vi "Test My Cloneable Module API.vi"() -> ()   [LabVIEW 2020]
doc: "My Module API Tester.\n_____\nBased on Delacor QMH Project Template 5.0.0.82."
uses:
  My Cloneable Module.lvlib
panel:
  in  "wait for reply":bool=TRUE
  in  "Run as Singleton?":bool
  in  "Show Block Diagram":bool
  in  "Refresh Modules":bool
  in  "X":dbl=1.0
  out "Reply Payload":dbl
  out "Active Modules":string[](array[string])
  in  "Stop Module":bool
  in  "Select Module":i32(ring)=-1 caption="Select Module\nTo send Request to" items=["All"=-1]
  in  "Run New Module":bool
  out "Do Something Count":i32
  in  "Test Do Something Else and Wait for Reply":bool
  in  "Hide Module Panel":bool
  in  "Show Module Panel":bool
  in  "Test Do Something Else":bool
  in  "Test Do Something":bool
  out "Status":string
  # "This VI tests the API for the Module."
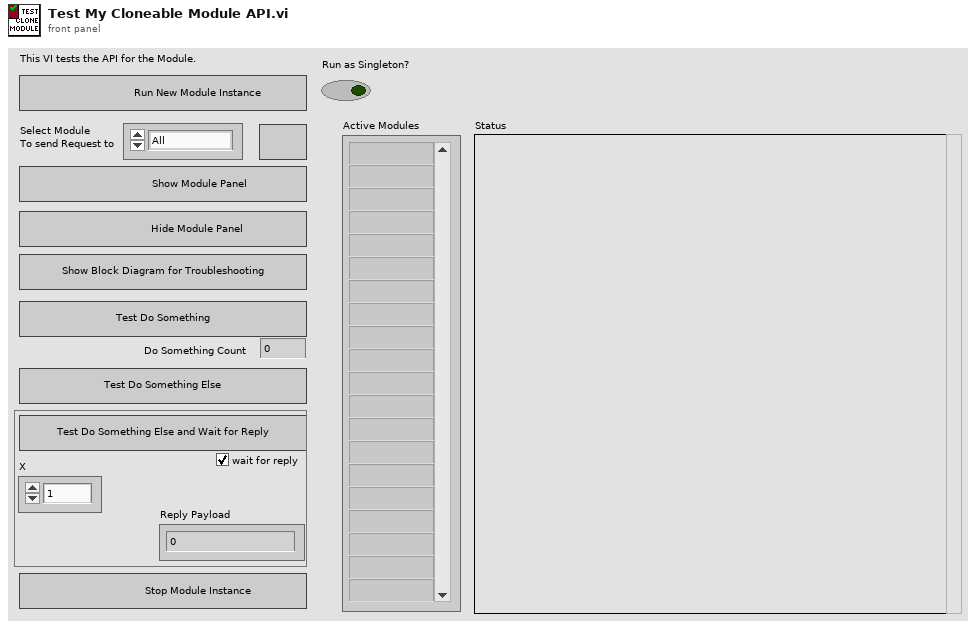
[diagram p1: front panel]
types:
  T1 = typedef "My Cloneable Module.lvlib/Broadcast Events--cluster.ctl" = cluster{"Module Did Init":refnum<user-event>, "Status Updated":refnum<user-event>, "Error Reported":refnum<user-event>, "Did Something":refnum<user-event>, "Module Did Stop":refnum<user-event>, "Update Module Execution Status":refnum<user-event>}
  T2 = typedef "My Cloneable Module.lvlib/Do Something Else and Wait (Reply Payload)--cluster.ctl" = cluster{"Value":dbl, "error":errorcluster}
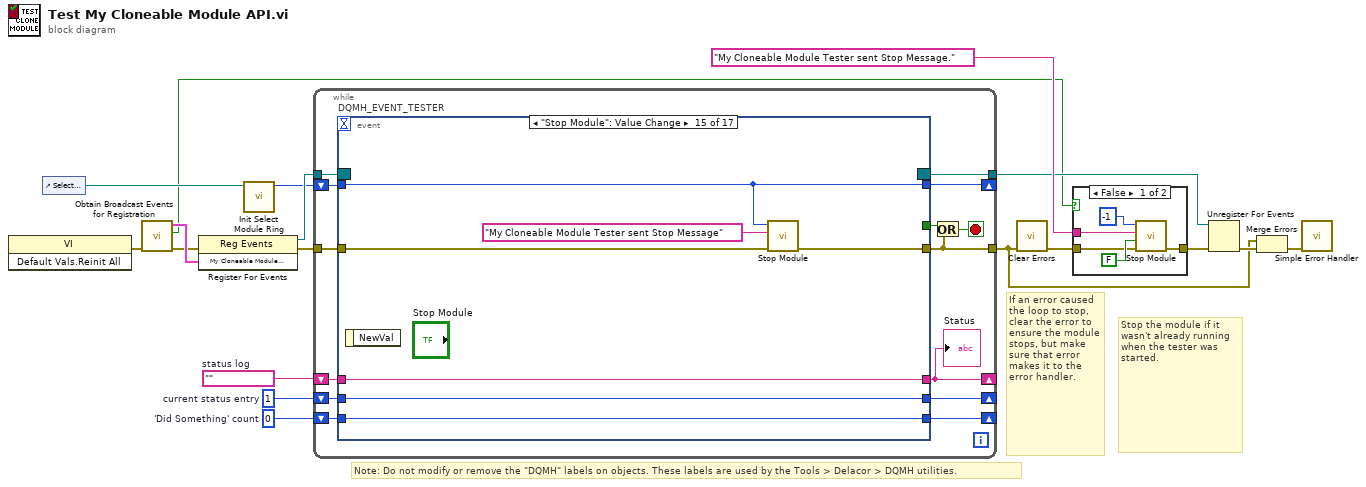
[diagram p0: block diagram]
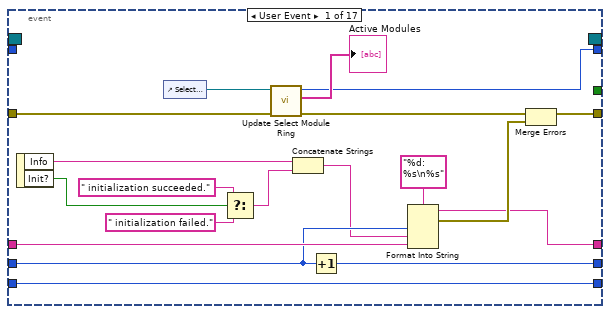
[diagram p3: hidden frame]
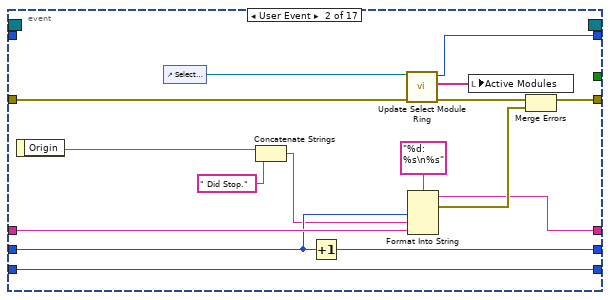
[diagram p4: hidden frame]
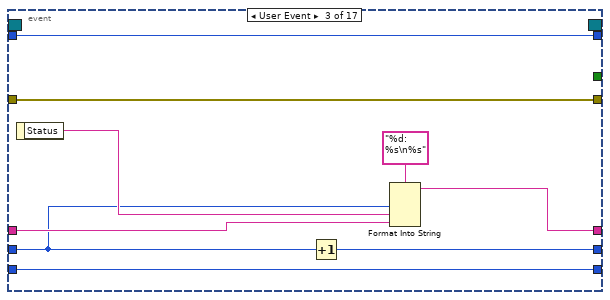
[diagram p5: hidden frame]
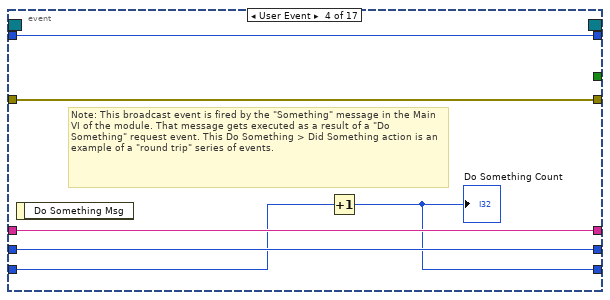
[diagram p6: hidden frame]
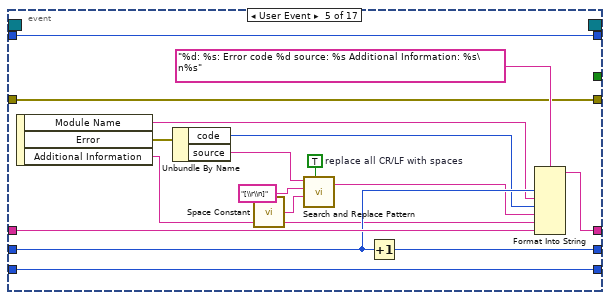
[diagram p7: hidden frame]
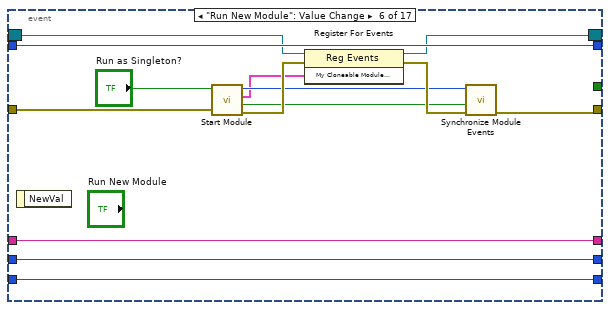
[diagram p8: hidden frame]
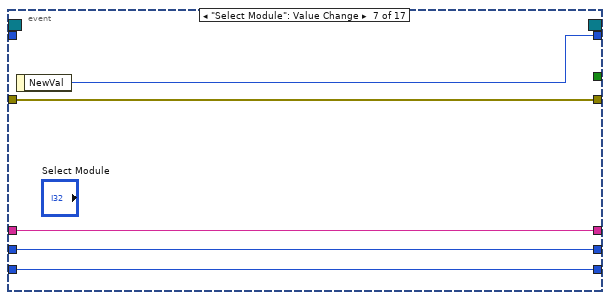
[diagram p9: hidden frame]
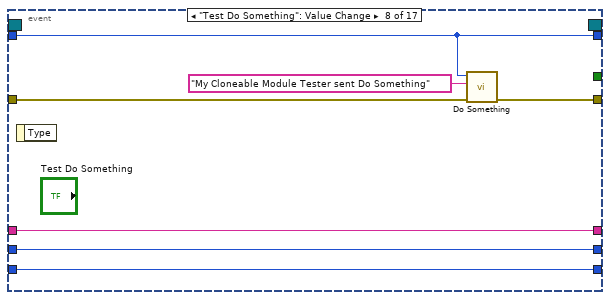
[diagram p10: hidden frame]
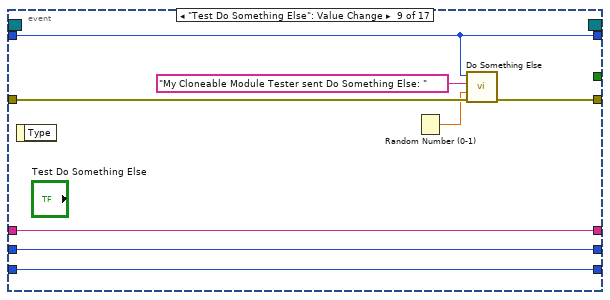
[diagram p11: hidden frame]
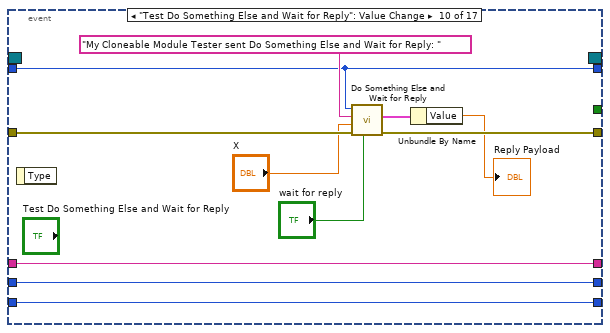
[diagram p12: hidden frame]
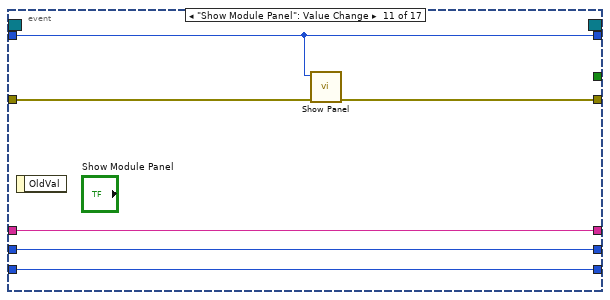
[diagram p13: hidden frame]
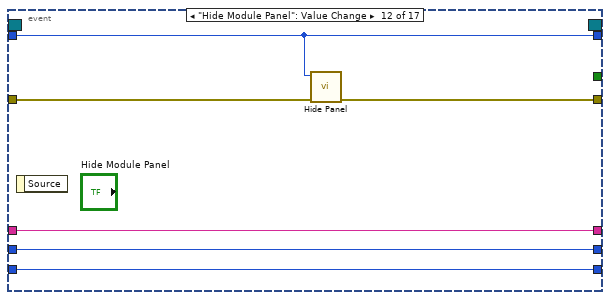
[diagram p14: hidden frame]
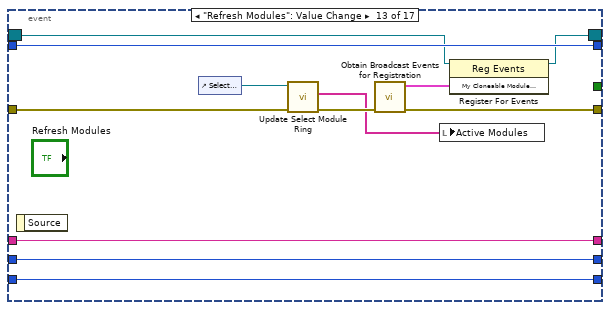
[diagram p15: hidden frame]
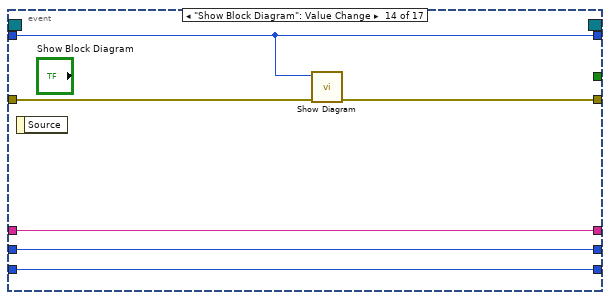
[diagram p16: hidden frame]
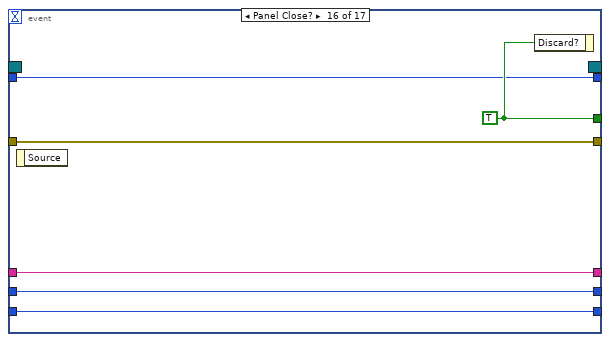
[diagram p17: hidden frame]
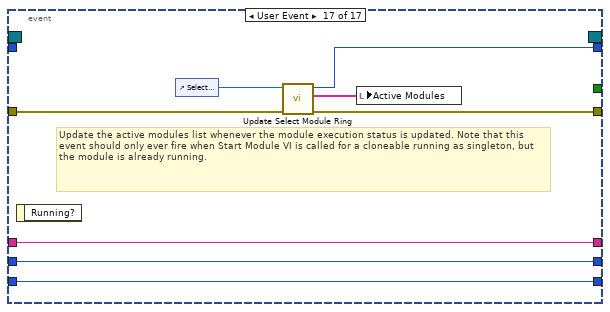
[diagram p18: hidden frame]
diagram:
  w13 = 0  # 'Did Something' count
  w14 = 1  # current status entry
  w15 = ""  # status log
  # "Stop the module if it wasn't already running when the tester was started."
  # "If an error caused the loop to stop, clear the error to ensure the module stops, but make sure that error makes it to the error handler."
  # "Note: Do not modify or remove the \"DQMH\" labels on objects. These labels are used by the Tools > Delacor > DQMH utilities."
  n1 = invoke class="VI" method="Default Vals.Reinit All"() -> (error out=w3:errorcluster)  [unwired: 3 in, 2 out]
  n2 = control-ref of="Select Module"() -> (w11:refnum<vi>)
  n3 = call "Obtain Broadcast Events for Registration.vi"("error in (no error)"=w3) -> ("error out"=w2:errorcluster, "Already running?"=w1:bool, "My Cloneable Module Broadcast Events"=w10:T1)  [unwired: 8 in]
  n4 = register-events(error in=w2, w10) -> (reference out=w18:refnum<event-registration>, error out=w9:errorcluster)  [unwired: 1 in]
  n5 = call "Init Select Module Ring.vi"("Select Module Ring Ref"=w11) -> ("Value for All Modules"=w12:i32)  [unwired: 8 in, 2 out]
  n6 = while {
    tunnel: w18 -> [w32]
    tunnel: [w19] -> w4
    tunnel: w9 -> [w30]
    shift-right: [w26] -> _
    shift-left: w15 -> [w28]
    shift-right: [w27] -> _
    shift-left: w14 -> [w29]
    shift-right: [w24] -> _
    shift-left: w13 -> [w25]
    shift-right: [w21] -> _
    shift-left: w12 -> [w22]
    tunnel: [w20] -> w7
    stop <- w23 stop-if-true
    n7 = event "DQMH_EVENT_TESTER" shown="[14] \"Stop Module\": Value Change" {
      selector: w32 -> [_ _ _ _ _ w106 _ _ _ _ _ _ w162 _ _ _ _]
      dyn-events: [_ _ _ _ _ w105 _ _ _ _ _ _ w161 _ _ _ _] -> w20
      timeout: _ -> [_ _ _ _ _ _ _ _ _ _ _ _ _ _ _ _ _]
      tunnel: [_ _ _ _ _ _ _ _ _ _ _ _ _ _ _ w187 _] -> w31
      tunnel: [w40 w58 w76 w82 w88 w104 w118 w124 w132 w144 w149 w155 w158 w170 w176 w186 w190] -> w19
      tunnel: w30 -> [w42 w60 w76 w82 w88 w107 w118 w125 w133 w136 w150 w156 w163 w174 w177 w186 w191]
      tunnel: w29 -> [w48 w64 w68 w80 w94 w110 w116 w121 w128 w141 w147 w153 w167 w172 w180 w184 w194]
      tunnel: w28 -> [w49 w65 w72 w81 w96 w111 w117 w122 w129 w142 w148 w154 w168 w173 w181 w185 w195]
      tunnel: [w46 w62 w73 w81 w91 w111 w117 w122 w129 w142 w148 w154 w168 w173 w181 w185 w195] -> w26
      tunnel: [w47 w63 w75 w80 w97 w110 w116 w121 w128 w141 w147 w153 w167 w172 w180 w184 w194] -> w27
      tunnel: w25 -> [w43 w61 w71 w79 w99 w109 w115 w120 w127 w140 w146 w152 w166 w171 w179 w183 w193]
      tunnel: [w43 w61 w71 w78 w99 w109 w115 w120 w127 w140 w146 w152 w166 w171 w179 w183 w193] -> w24
      tunnel: w22 -> [_ _ w69 w77 w98 w108 _ w119 w126 w139 w145 w151 w165 w169 w178 w182 _]
      tunnel: [w37 w55 w69 w77 w98 w108 w114 w119 w126 w139 w145 w151 w165 w169 w178 w182 w189] -> w21
      event User Event {
        n8 = event-data() -> ("Info"=w45:string, "Init?"=w34:bool)  [unwired: 1 in]
        n9 = control-ref of="Select Module"() -> (w39:refnum<vi>)
        n10 = Select(t=" initialization succeeded.", s=w34, f=" initialization failed.") -> (s? t:f=w33:string)
        n11 = call "Update Select Module Ring.vi"("error in (no error)"=w42, "Select Module Ring Ref"=w39) -> ("error out"=w41:errorcluster, "Active Modules (Array)"=→"Active Modules":string[], "New Module Ring Value"=w37:i32)  [unwired: 7 in]
        n12 = Concatenate Strings(w45, w33) -> (w44:string)
        n13 = Increment(x=w48) -> (x+1=w47:i32)
        n14 = Format Into String(format string="%d: %s\n%s", w48, w44, w49) -> (resulting string=w46:string, error out=w51:errorcluster)  [unwired: 2 in]
        n15 = Merge Errors(w41, w51) -> (w40:errorcluster)
      }
      event User Event {
        n16 = event-data() -> ("Origin"=w53:string)  [unwired: 1 in]
        n17 = control-ref of="Select Module"() -> (w57:refnum<vi>)
        n18 = Concatenate Strings(w53, " Did Stop.") -> (w52:string)
        n19 = Increment(x=w64) -> (x+1=w63:i32)
        n20 = call "Update Select Module Ring.vi"("error in (no error)"=w60, "Select Module Ring Ref"=w57) -> ("error out"=w59:errorcluster, "Active Modules (Array)"=w56:string[], "New Module Ring Value"=w55:i32)  [unwired: 7 in]
        n21 = Format Into String(format string="%d: %s\n%s", w64, w52, w65) -> (resulting string=w62:string, error out=w67:errorcluster)  [unwired: 2 in]
        n22 = local write "Active Modules"(w56) -> ()
        n23 = Merge Errors(w59, w67) -> (w58:errorcluster)
      }
      event User Event {
        n24 = event-data() -> ("Status"=w70:string)  [unwired: 1 in]
        n25 = Increment(x=w68) -> (x+1=w75:i32)
        n26 = Format Into String(format string="%d: %s\n%s", w68, w70, w72) -> (resulting string=w73:string)  [unwired: 2 in, 1 out]
      }
      event User Event {
        # "Note: This broadcast event is fired by the \"Something\" message in the Main VI of the module. That message gets executed as a result of a \"Do Something\" request event. This Do Something > Did Something action is an example of a \"round trip\" series of events."
        n27 = event-data() -> ()  [unwired: 1 in, 1 out]
        n28 = Increment(x=w79) -> (x+1=w78:i32)
        "Do Something Count" <- w78
      }
      event User Event {
        w92 = TRUE  # replace all CR/LF with spaces
        n29 = event-data() -> ("Module Name"=w86:string, "Error"=w85:errorcluster, "Additional Information"=w83:string)  [unwired: 1 in]
        n30 = Unbundle By Name(w85) -> ("code"=w87:i32, "source"=w89:string)
        n31 = call <vilib>:"Space Constant.vi"() -> ("String"=w93:string)
        n32 = call <vilib>:"Search and Replace Pattern.vi"("string"=w89, "regular expression (\"\")"="[\\r\\n]" ("regular expression (\"\")"), "replace string (\"\")"=w93, "replace all? (F)"=w92) -> ("result string"=w90:string)  [unwired: 1 in, 1 out]
        n33 = Increment(x=w94) -> (x+1=w97:i32)
        n34 = Format Into String(format string="%d: %s: Error code %d source: %s Additional Information: %s\n%s", w94, w86, w87, w90, w83, w96) -> (resulting string=w91:string)  [unwired: 2 in, 1 out]
      }
      event "Run New Module": Value Change {
        n35 = event-data() -> ()  [unwired: 1 in, 1 out]
        n36 = call "Start Module.vi"("error in (no error)"=w107, "Run as Singleton? (F)"="Run as Singleton?") -> ("error out"=w112:errorcluster, "Wait for Event Sync?"=w102:bool, "My Cloneable Module Broadcast Events"=w101:T1, "Module ID"=w103:i32)  [unwired: 6 in]
        n37 = register-events(reference=w106, error in=w112, w101) -> (reference out=w105:refnum<event-registration>, error out=w113:errorcluster)
        n38 = call "Synchronize Module Events.vi"("error in (no error)"=w113, "Wait for Event Sync?"=w102, "Module ID"=w103) -> ("error out"=w104:errorcluster)  [unwired: 7 in, 1 out]
      }
      event "Select Module": Value Change {
        n39 = event-data() -> ("NewVal"=w114:i32)  [unwired: 1 in]
      }
      event "Test Do Something": Value Change {
        n40 = event-data() -> ()  [unwired: 1 in, 1 out]
        n41 = call "Do Something.vi"("error in (no error)"=w125, "Do Something Message"="My Cloneable Module Tester sent Do Something", "Module ID"=w119) -> ("error out"=w124:errorcluster)  [unwired: 8 in]
      }
      event "Test Do Something Else": Value Change {
        n42 = event-data() -> ()  [unwired: 1 in, 1 out]
        n43 = Random Number (0-1)() -> (number: 0 to 1=w130:dbl)
        n44 = call "Do Something Else.vi"("error in (no error)"=w133, "X"=w130, "Do Something else Message"="My Cloneable Module Tester sent Do Something Else: " ("Do Something Message"), "Module ID"=w126) -> ("error out"=w132:errorcluster)  [unwired: 7 in]
      }
      event "Test Do Something Else and Wait for Reply": Value Change {
        n45 = event-data() -> ()  [unwired: 1 in, 1 out]
        n46 = call "Do Something Else and Wait for Reply.vi"("wait for reply (T)"="wait for reply", "error in (no error)"=w136, "X"="X", "Do Something Else Message"="My Cloneable Module Tester sent Do Something Else and Wait for Reply: " ("Do Something Message"), "Module ID"=w139) -> ("error out"=w144:errorcluster, "Reply Payload"=w138:T2)  [unwired: 4 in, 1 out]
        n47 = Unbundle By Name(w138) -> ("Value"=→"Reply Payload":dbl)
      }
      event "Show Module Panel": Value Change {
        n48 = event-data() -> ()  [unwired: 1 in, 1 out]
        n49 = call "Show Panel.vi"("error in (no error)"=w150, "Module ID"=w145) -> ("error out"=w149:errorcluster)  [unwired: 9 in]
      }
      event "Hide Module Panel": Value Change {
        n50 = event-data() -> ()  [unwired: 1 in, 1 out]
        n51 = call "Hide Panel.vi"("error in (no error)"=w156, "Module ID"=w151) -> ("error out"=w155:errorcluster)  [unwired: 9 in]
      }
      event "Refresh Modules": Value Change {
        n52 = event-data() -> ()  [unwired: 1 in, 1 out]
        n53 = control-ref of="Select Module"() -> (w164:refnum<vi>)
        n54 = call "Update Select Module Ring.vi"("error in (no error)"=w163, "Select Module Ring Ref"=w164) -> ("error out"=w159:errorcluster, "Active Modules (Array)"=w157:string[])  [unwired: 7 in, 1 out]
        n55 = call "Obtain Broadcast Events for Registration.vi"("error in (no error)"=w159) -> ("error out"=w158:errorcluster, "My Cloneable Module Broadcast Events"=w160:T1)  [unwired: 8 in, 1 out]
        n56 = local write "Active Modules"(w157) -> ()
        n57 = register-events(reference=w162, w160) -> (reference out=w161:refnum<event-registration>)  [unwired: 1 in, 1 out]
      }
      event "Show Block Diagram": Value Change {
        n58 = event-data() -> ()  [unwired: 1 in, 1 out]
        n59 = call "Show Diagram.vi"("error in (no error)"=w174, "Module ID"=w169) -> ("error out"=w170:errorcluster)  [unwired: 9 in]
      }
      event "Stop Module": Value Change {
        n60 = event-data() -> ()  [unwired: 1 in, 1 out]
        n61 = call "Stop Module.vi"("error in (no error)"=w177, "Origin"="My Cloneable Module Tester sent Stop Message", "Module ID"=w178) -> ("error out"=w176:errorcluster)  [unwired: 8 in]
      }
      event Panel Close? {
        w187 = TRUE ("Discard?")
        n62 = event-data() -> ()  [unwired: 1 in, 1 out]
        n63 = event-data("Discard?"=w187) -> ()  [unwired: 1 in, 1 out]
      }
      event User Event {
        # "Update the active modules list whenever the module execution status is updated. Note that this event should only ever fire when Start Module VI is called for a cloneable running as singleton, but the module is already running."
        n64 = event-data() -> ()  [unwired: 1 in, 1 out]
        n65 = control-ref of="Select Module"() -> (w192:refnum<vi>)
        n66 = call "Update Select Module Ring.vi"("error in (no error)"=w191, "Select Module Ring Ref"=w192) -> ("error out"=w190:errorcluster, "Active Modules (Array)"=w188:string[], "New Module Ring Value"=w189:i32)  [unwired: 7 in]
        n67 = local write "Active Modules"(w188) -> ()
      }
    }
    "Status" <- w26
    n68 = Or(x=w31, y=w19) -> (x .or. y?=w23:bool)
  }
  n69 = call <vilib>:"Clear Errors.vi"("error in (no error)"=w4) -> ("error out"=w6:errorcluster)  [unwired: 5 in, 1 out]
  n70 = case shown="False" w1 {
    tunnel: [w200 w201] -> w16
    tunnel: "My Cloneable Module Tester sent Stop Message." ("Origin") -> [w199 _]
    tunnel: w6 -> [w196 w201]
    frame False {
      n71 = call "Stop Module.vi"("error in (no error)"=w196, "Wait for Module to stop? (F)"=FALSE ("Wait for Module to stop?"), "Origin"=w199, "Module ID"=-1 ("Stop all")) -> ("error out"=w200:errorcluster)  [unwired: 7 in]
    }
    frame True {
    }
  }
  n72 = Unregister For Events(event registration refnum=w7, error in=w16) -> (error out=w17:errorcluster)
  n73 = Merge Errors(w4, w17) -> (w5:errorcluster)
  n74 = call <vilib>:"Simple Error Handler.vi"("error in (no error)"=w5) -> ()  [unwired: 4 in, 5 out]
